vi "se2.vi"(6 "angle unit":u16(ring) items=["radians", "degrees"], 8 "error in (no error)":errorcluster, 9 "theta":dbl, 10 "y":dbl, 11 "x":dbl) -> (0 "Error Out":errorcluster, 3 "T":dbl[][](array[numeric]))   [LabVIEW 2017]
doc: "This function builds and outputs a 3x3 homogeneous transformation as a 2-D array(T). Inputs are horizontal translation (X), vertical translation (Y), and rotation (theta) in radians. The default value of theta is 0 rad."
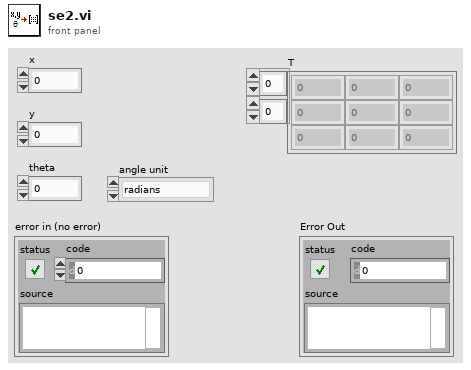
[diagram p1: front panel]
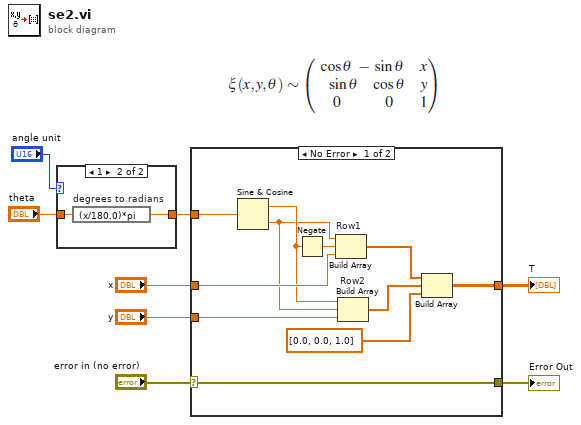
[diagram p0: block diagram]
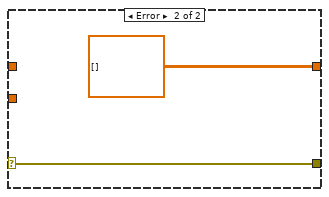
[diagram p3: hidden frame]
diagram:
  n1 = case shown="1" "angle unit" {
    tunnel: "theta" -> [w9 w11]
    tunnel: [w9 w10] -> w2
    frame 0, Default {
    }
    frame 1 {
      n2 = expression code="(x/180.0)*pi" "degrees to radians"(w11) -> (w10:dbl)
    }
  }
  n3 = case shown="No Error" "error in (no error)" {
    selector: "error in (no error)" -> [w22 w23]
    tunnel: [w22 w23] -> w7
    tunnel: "x" -> [w21 _]
    tunnel: "y" -> [w19 _]
    tunnel: w2 -> [w14 _]
    tunnel: [w15 dbl[][] [] ("t")] -> w4
    frame No Error {
      n4 = Sine & Cosine(0:w14) -> (1:w20:dbl, 2:w12:dbl)
      n5 = Negate(x=w20) -> (-x=w13:dbl)
      n6 = Build Array "Row1"(w12, w13, w21) -> (w18:dbl[])
      n7 = Build Array "Row2"(w20, w12, w19) -> (w17:dbl[])
      n8 = Build Array(w18, w17, dbl[] [0.0, 0.0, 1.0] ("appended array")) -> (w15:dbl[][])
    }
    frame Error {
    }
  }
  "Error Out" <- w7
  "T" <- w4
